vi "Modify Project.vi"(5 "Description":string, 7 "Creator":string, 8 "error in (no error)":errorcluster, 10 "Name":string, 11 "Project Root Path":path) -> (0 "error out":errorcluster, 1 "Project Path":path, 2 "Name out":string, 3 "Project Root Path dup":path)   [LabVIEW 2013, in "Project Wizard.lvlib"]
uses:
  Project Wizard.lvlib
  NationalInstruments.VeriStand.SystemStorage
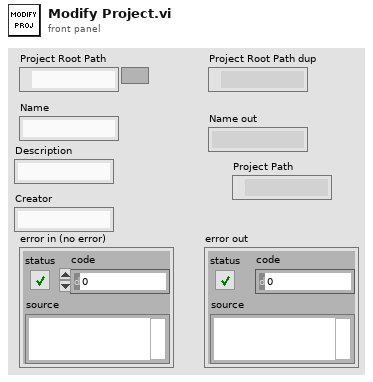
[diagram p1: front panel]
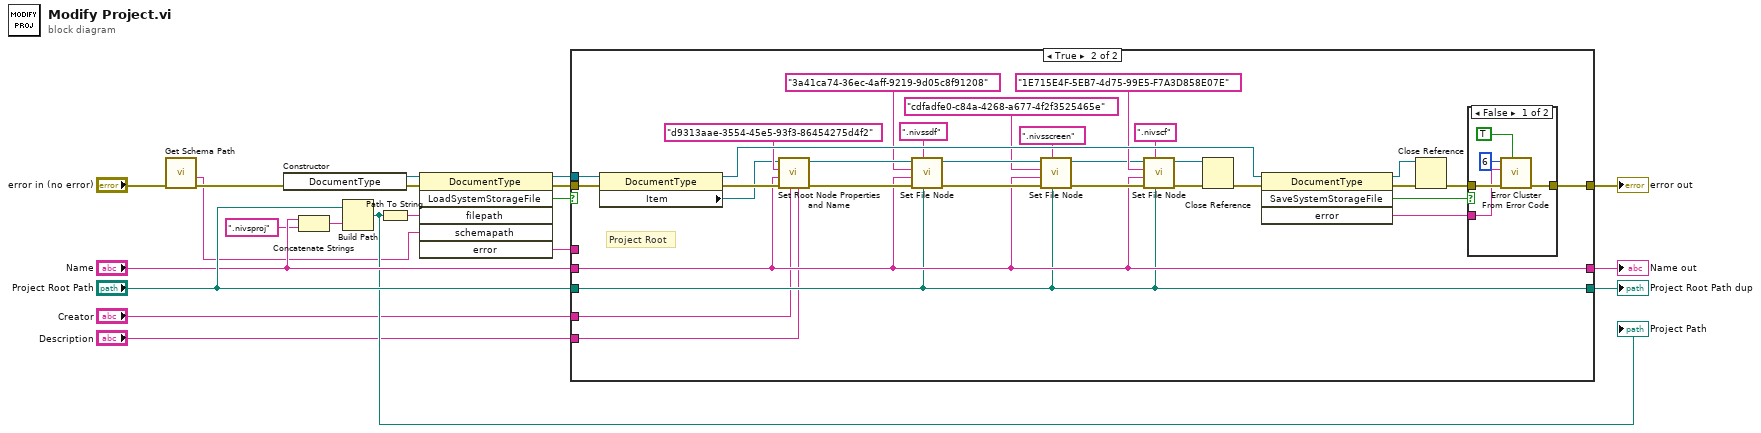
[diagram p0: block diagram]
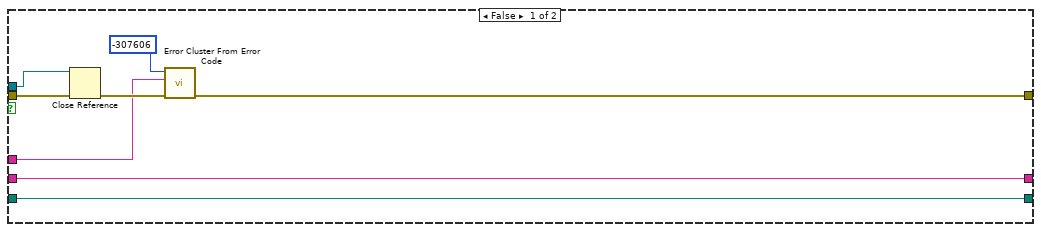
[diagram p2: hidden frame]
diagram:
  n1 = call "Get Schema Path.vi"("error in (no error)"="error in (no error)") -> ("error out"=w4:errorcluster, "Schema Path"=w3:string)  [unwired: 9 in]
  n2 = constructor class="DocumentType"(error in=w4) -> (reference out=w11:refnum<k24>, error out=w12:errorcluster)  [unwired: 2 in, 1 out]
  n3 = Concatenate Strings("Name", ".nivsproj" ("string")) -> (w6:string)
  n4 = Build Path(base path="Project Root Path", name or relative path=w6) -> (appended path=w14:path)
  "Project Path" <- w14
  n5 = Path To String(path=w14) -> (string=w13:string)
  n6 = invoke class="DocumentType" method="LoadSystemStorageFile"(reference=w11, error in=w12, "filepath"=w13, "schemapath"=w3) -> (reference out=w10:refnum<k24>, error out=w9:errorcluster, "LoadSystemStorageFile"=w8:bool, "error"=w7:string)  [unwired: 2 in, 2 out]
  n7 = case shown="True" w8 {
    tunnel: w10 -> [w28 w59]
    tunnel: w9 -> [w27 w58]
    tunnel: "Name" -> [w22 w36]
    tunnel: [w23 w31] -> w20
    tunnel: w7 -> [w25 _]
    tunnel: "Project Root Path" -> [w21 w35]
    tunnel: [w22 w36] -> w17
    tunnel: [w21 w35] -> w16
    tunnel: "Creator" -> [_ w30]
    tunnel: "Description" -> [_ w29]
    frame False {
      n8 = Close Reference(reference=w28, error in (no error)=w27) -> (error out=w26:errorcluster)
      n9 = call <vilib>:"Error Cluster From Error Code.vi"("error in (no error)"=w26, "error message (\"\")"=w25, "error code (0)"=-307606) -> ("error out"=w23:errorcluster)  [unwired: 6 in]
    }
    frame True {
      # "Project Root"
      n10 = property class="DocumentType"(reference=w59, error in=w58) -> (reference out=w55:refnum<k24>, error out=w52:errorcluster, "Item"=w51:refnum<k24>)
      n11 = call "Set Root Node Properties and Name.vi"("Description"=w29, "Creator"=w30, "error in (no error)"=w52, "Name"=w36, "guid"="d9313aae-3554-45e5-93f3-86454275d4f2", "Doc in"=w51) -> ("error out"=w50:errorcluster, "Doc out"=w49:refnum<k24>)  [unwired: 4 in]
      n12 = call "Set File Node.vi"("Path"=w35, "Extension"=".nivssdf" ("string"), "error in (no error)"=w50, "Name"=w36, "guid"="3a41ca74-36ec-4aff-9219-9d05c8f91208", "Doc in"=w49) -> ("error out"=w46:errorcluster, "Doc out"=w45:refnum<k24>)  [unwired: 4 in]
      n13 = call "Set File Node.vi"("Path"=w35, "Extension"=".nivsscreen" ("string"), "error in (no error)"=w46, "Name"=w36, "guid"="cdfadfe0-c84a-4268-a677-4f2f3525465e", "Doc in"=w45) -> ("error out"=w40:errorcluster, "Doc out"=w39:refnum<k24>)  [unwired: 4 in]
      n14 = call "Set File Node.vi"("Path"=w35, "Extension"=".nivscf" ("string"), "error in (no error)"=w40, "Name"=w36, "guid"="1E715E4F-5EB7-4d75-99E5-F7A3D858E07E", "Doc in"=w39) -> ("error out"=w37:errorcluster, "Doc out"=w38:refnum<k24>)  [unwired: 4 in]
      n15 = Close Reference(reference=w38, error in (no error)=w37) -> (error out=w57:errorcluster)
      n16 = invoke class="DocumentType" method="SaveSystemStorageFile"(reference=w55, error in=w57) -> (reference out=w54:refnum<k24>, error out=w56:errorcluster, "SaveSystemStorageFile"=w34:bool, "error"=w32:string)  [unwired: 2 in]
      n17 = Close Reference(reference=w54, error in (no error)=w56) -> (error out=w33:errorcluster)
      n18 = case shown="False" w34 {
        tunnel: w33 -> [w64 w65]
        tunnel: w32 -> [w63 _]
        tunnel: [w60 w65] -> w31
        frame False {
          n19 = call <vilib>:"Error Cluster From Error Code.vi"("show call chain? (False)"=TRUE, "error in (no error)"=w64, "error message (\"\")"=w63, "error code (0)"=6) -> ("error out"=w60:errorcluster)  [unwired: 5 in]
        }
        frame True {
        }
      }
    }
  }
  "error out" <- w20
  "Project Root Path dup" <- w16
  "Name out" <- w17
